vi "Initialise Channel.vi"(5 "Data Format In":T16 {"Coupling Level" max=4095 step=1}, 6 "Channel In":T19(ring), 7 "Gates In":T12 {"Gate 4"."Max # Peaks" max=64000 step=100; "Gate 4"."Threshold" min=10 max=4095 step=10; "Gate 4"."Length (us)" min=0.0 max=96000.0 step=100.0; "Gate 4"."Start (us)" min=0.0 max=64000.0 step=100.0; "Gate 3"."Max # Peaks" max=64000 step=100; "Gate 3"."Threshold" min=10 max=4095 step=10; "Gate 3"."Length (us)" min=0.0 max=96000.0 step=100.0; "Gate 3"."Start (us)" min=0.0 max=64000.0 step=100.0; "Gate 2"."Max # Peaks" max=64000 step=100; "Gate 2"."Threshold" min=10 max=4095 step=10; "Gate 2"."Length (us)" min=0.0 max=96000.0 step=100.0; "Gate 2"."Start (us)" min=0.0 max=64000.0 step=100.0; "Gate 1"."Max # Peaks" max=64000 step=100; "Gate 1"."Threshold" min=10 max=4095 step=10; "Gate 1"."Length (us)" min=0.0 max=96000.0 step=100.0; "Gate 1"."Start (us)" min=0.0 max=64000.0 step=100.0}, 8 "error in (no error)":errorcluster, 9 "Transmit In (TX)":T9 {"Pulse Shape"."Width" min=16 max=1010 step=50 format="%.0fns"}, 10 "Recieve In (RX)":T1 {"Delay" min=0.0 format="%#_g us"; "Display Gate"."Length" min=0.0 max=64000.0 step=1.0 format="%#_g us"; "Display Gate"."Start" min=0.0 max=64000.0 step=1.0 format="%#_g us"; "Analogue Filtering"."Smoothing" min=1 max=11 step=1; "Gain" min=-6.0 max=70.0 step=0.25 format="%.2fdB"}, 11 "Test Reference In":refnum<vi>) -> (0 "error out":errorcluster)   [LabVIEW 2026]
uses:
  <instrlib>/MicroPulse/MicroPulse_Driver.lvlib
  <instrlib>/MicroPulse/Public/Data/Datatypes/MP - amplitude reporting mode.ctl
  <instrlib>/MicroPulse/Public/Data/Datatypes/MP - averaging.ctl
  <instrlib>/MicroPulse/Public/Data/Datatypes/MP - data formatting.ctl
  <instrlib>/MicroPulse/Public/Data/Datatypes/MP - hysteresis level.ctl
  <instrlib>/MicroPulse/Public/Data/Datatypes/MP - multigate mode.ctl
  <instrlib>/MicroPulse/Public/Data/Datatypes/MP - multigate inspection gate parameters.ctl
  <instrlib>/MicroPulse/Public/Data/Datatypes/MP - multi-gate inspection.ctl
  <instrlib>/MicroPulse/Public/Data/Datatypes/MP - pulser voltage.ctl
  <instrlib>/MicroPulse/Public/Data/Datatypes/MP - pulse damping.ctl
  <instrlib>/MicroPulse/Public/Data/Datatypes/MP - transmit parameters.ctl
  <instrlib>/MicroPulse/Public/Data/Datatypes/MP - waveform type.ctl
  <instrlib>/MicroPulse/Public/Data/Datatypes/MP - frequency filter.ctl
  <instrlib>/MicroPulse/Public/Data/Datatypes/MP - analogue filter.ctl
  <instrlib>/MicroPulse/Public/Data/Datatypes/MP - high pass filter.ctl
  <instrlib>/MicroPulse/Public/Data/Datatypes/MP - low pass filter.ctl
  <instrlib>/MicroPulse/Public/Data/Datatypes/MP - digital filtering.ctl
  <instrlib>/MicroPulse/Public/Data/Datatypes/MP - display gate.ctl
  <instrlib>/MicroPulse/Public/Data/Datatypes/MP - receive parameters.ctl
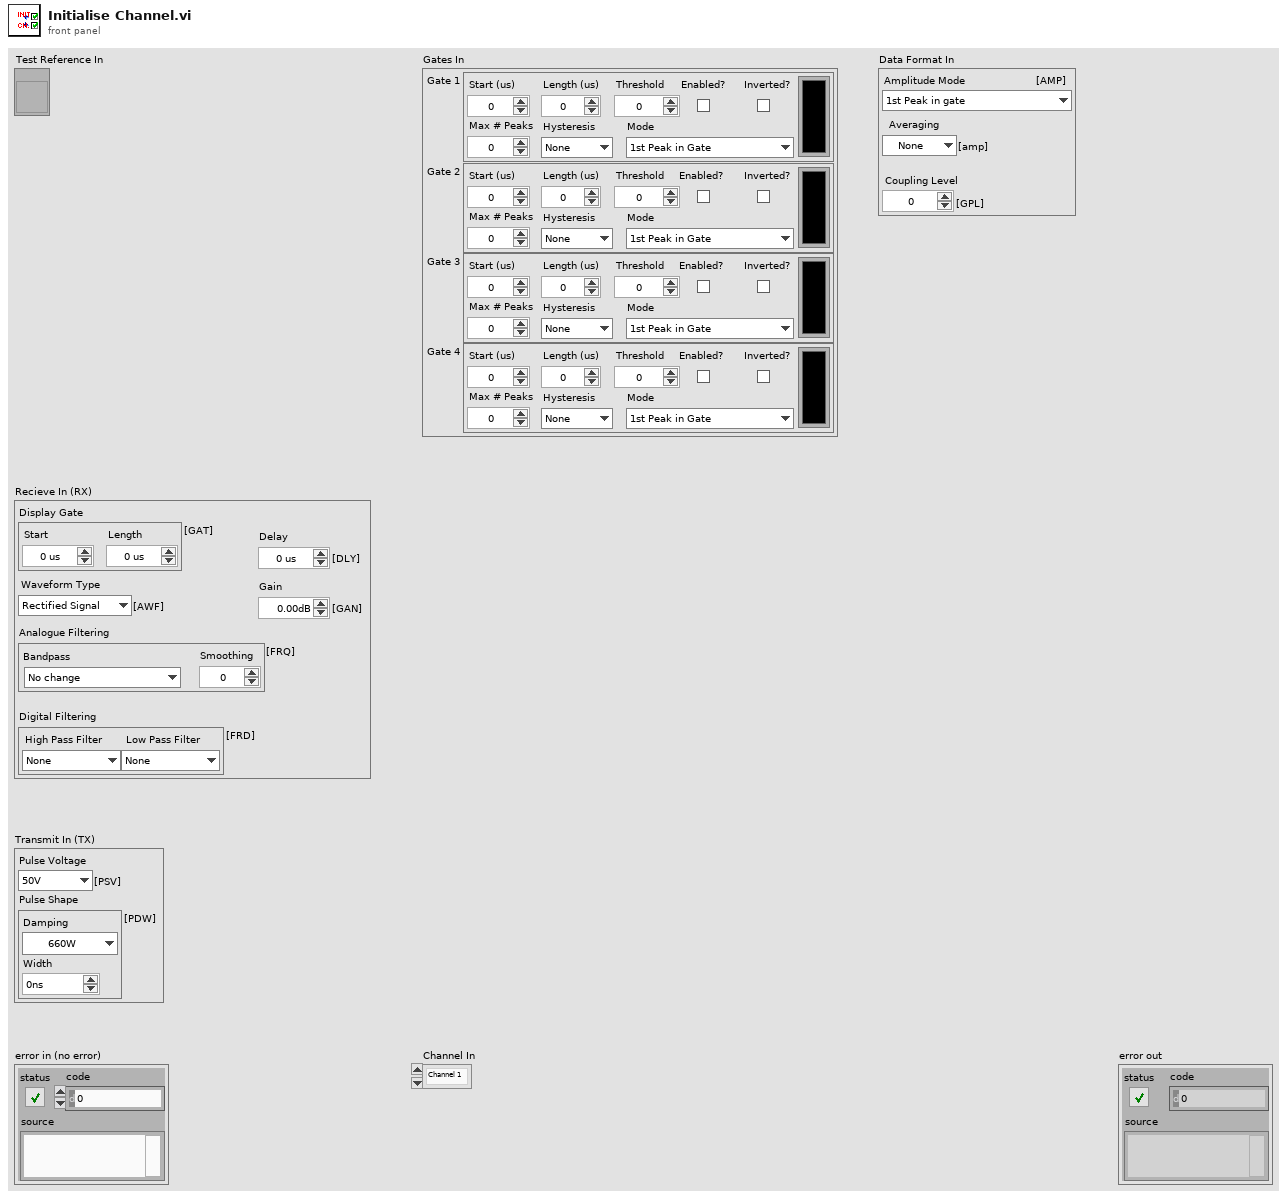
[diagram p1: front panel]
types:
  T1 = typedef "MicroPulse_Driver.lvlib/MP - receive parameters.ctl" = cluster{"Display Gate":T2, "Delay":dbl, "Waveform Type":T3, "Gain":dbl, "Analogue Filtering":T4, "Digital Filtering":T6}
  T2 = typedef "MicroPulse_Driver.lvlib/MP - display gate.ctl" = cluster{"Start":dbl, "Length":dbl}
  T3 = typedef "MicroPulse_Driver.lvlib/MP - waveform type.ctl" = enum16{"Rectified Signal", "RF Signal", "+Half Wave", "-Half Wave"}
  T4 = typedef "MicroPulse_Driver.lvlib/MP - analogue filter.ctl" = cluster{"Bandpass":T5, "Smoothing":u16}
  T5 = typedef "MicroPulse_Driver.lvlib/MP - frequency filter.ctl" = enum16{"No change", "1MHz Bandpass", "2MHz Bandpass", "4MHz Bandpass", "5MHz Bandpass", "10MHz Bandpass", "2.5-18MHz Broadband", "0.75-12MHz  Broadband", "0.5MHz Bandpass", "5MHz 2nd Order TOFD", "10MHz 2nd Order TOFD", "3.0-25MHz Broadband", "3.0-30MHz Broadband"}
  T6 = typedef "MicroPulse_Driver.lvlib/MP - digital filtering.ctl" = cluster{"High Pass Filter":T7, "Low Pass Filter":T8}
  T7 = typedef "MicroPulse_Driver.lvlib/MP - high pass filter.ctl" = enum16{"None", "0.7MHz", "1.5MHz", "4.0MHz", "7.5MHz", "10.0MHz", "User Defined"}
  T8 = typedef "MicroPulse_Driver.lvlib/MP - low pass filter.ctl" = enum16{"None", "1.8MHz", "3.0MHz", "6.0MHz", "8.0MHz", "12.0MHz", "User Defined"}
  T9 = typedef "MicroPulse_Driver.lvlib/MP - transmit parameters.ctl" = cluster{"Pulse Voltage":T10, "Pulse Shape":cluster{"Damping":T11, "Width":u32}}
  T10 = typedef "MicroPulse_Driver.lvlib/MP - pulser voltage.ctl" = enum16{"50V", "100V", "150V", "200V", "250V", "300V"}
  T11 = typedef "MicroPulse_Driver.lvlib/MP - pulse damping.ctl" = enum16{"660W", "458W", "220W", "149W", "102W", "82W", "63W", "51W"}
  T12 = typedef "MicroPulse_Driver.lvlib/MP - multi-gate inspection.ctl" = cluster{"Gate 1":T13, "Gate 2":T13, "Gate 3":T13, "Gate 4":T13}
  T13 = typedef "MicroPulse_Driver.lvlib/MP - multigate inspection gate parameters.ctl" = cluster{"Start (us)":dbl, "Length (us)":dbl, "Threshold":u16, "Enabled?":bool, "Max # Peaks":u16, "Hysteresis":T14, "Mode":T15, "Inverted?":bool, "Colour ":u32}
  T14 = typedef "MicroPulse_Driver.lvlib/MP - hysteresis level.ctl" = enum16{"None", "3dB", "6dB", "9dB", "12dB"}
  T15 = typedef "MicroPulse_Driver.lvlib/MP - multigate mode.ctl" = enum16{"1st Peak in Gate", "Largest Peak In Gate", "All Peaks In Gate", "1st Threshold Crossing"}
  T16 = typedef "MicroPulse_Driver.lvlib/MP - data formatting.ctl" = cluster{"Amplitude Mode":T17, "Averaging":T18, "Coupling Level":u32}
  T17 = typedef "MicroPulse_Driver.lvlib/MP - amplitude reporting mode.ctl" = enum16{"1st Peak in gate", "Maximum Peak in gate", "All Peaks", "Ascan Data", "1st Threshold Crossing Peak", "Ascan + Peaks", "All Peaks for Multigate", "Peaks + Ascan for Multigate", "Peaks + P_Ascan for Multigate", "Full Matrix Capture"}
  T18 = typedef "MicroPulse_Driver.lvlib/MP - averaging.ctl" = enum16{"None", "2", "4", "8", "16", "32", "64", "128", "256"}
  T19 = enum16{"Channel 1", "Channel 2", "Channel 3", "Channel 4", "Channel 5", "Channel 6", "Channel 7"}
  T20 = typedef "MicroPulse_Driver.lvlib/MP - test parameters.ctl" = cluster{"Test No.":u32, "Tx Channel":u32, "Rx Channel":u32}
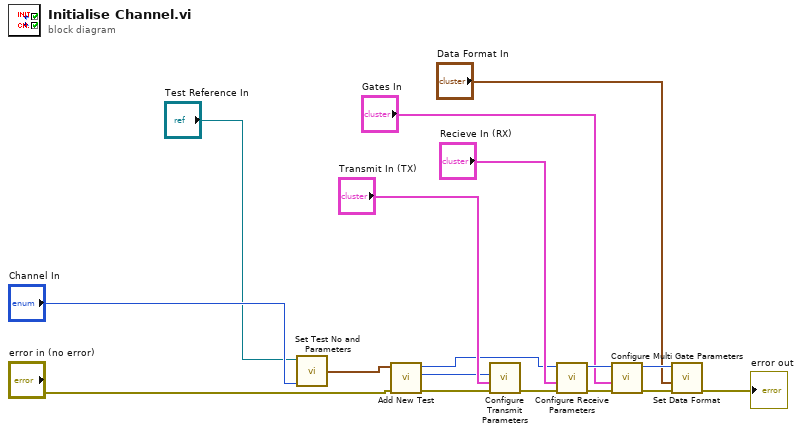
[diagram p0: block diagram]
diagram:
  n1 = call "Set Test No and Parameters.vi"("Channel Select"="Channel In", "Test Parameters In"="Test Reference In") -> ("Test Parameters Out"=w17:T20)  [unwired: 4 in]
  n2 = call <instrlib>:"Add New Test.vi"("error in (no error)"="error in (no error)", "Test Parameters"=w17) -> ("error out"=w3:errorcluster, "Tx Channel out"=w2:u32, "Test No. out"=w4:u32)  [unwired: 6 in, 1 out]
  n3 = call <instrlib>:"Configure Transmit Parameters.vi"("error in (no error)"=w3, "Transmit Parameters"="Transmit In (TX)", "Tx Channel"=w2) -> ("error out"=w7:errorcluster)  [unwired: 7 in, 1 out]
  n4 = call <instrlib>:"Configure Receive Parameters.vi"("error in (no error)"=w7, "Receive Parameters"="Recieve In (RX)", "Test No."=w4) -> ("error out"=w10:errorcluster, "Test No. out"=w9:u32)  [unwired: 6 in, 1 out]
  n5 = call <instrlib>:"Configure Multi Gate Parameters.vi"("error in (no error)"=w10, "Multi Gate Inspection"="Gates In", "Test Number"=w9) -> ("error out"=w13:errorcluster, "Test Number out"=w12:u32)  [unwired: 6 in, 1 out]
  n6 = call <instrlib>:"Set Data Format.vi"("error in (no error)"=w13, "Data Formatting"="Data Format In", "Test No."=w12) -> ("error out"=→"error out":errorcluster)  [unwired: 6 in, 2 out]
